vi "Read Graph Properties.vi"(0 "Config File":path, 7 "WFGraph Refnum":refnum<vi>, 9 "Section":string, 11 "error in (no error)":errorcluster) -> (4 "Config File out":path, 15 "error out":errorcluster)   [LabVIEW 2020]
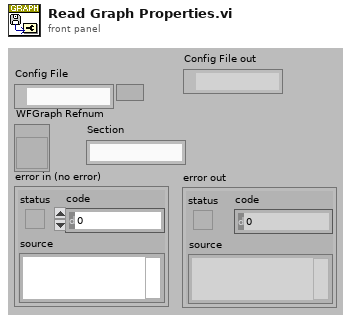
[diagram p1: front panel]
types:
  T1 = typedef "Graph Properties.ctl" = cluster{"X-axis":T2, "Y-axis":T2, "Plot Properties":T3[]}
  T2 = typedef "Axis Properties.ctl" = cluster{"Min":dbl, "Max":dbl, "Fit":u8}
  T3 = typedef "Plot Properties.ctl" = cluster{"Line Style":u8, "Line Width":u8, "Plot Color":u32, "Point Style":u8, "Point color":u32, "Interp":u8}
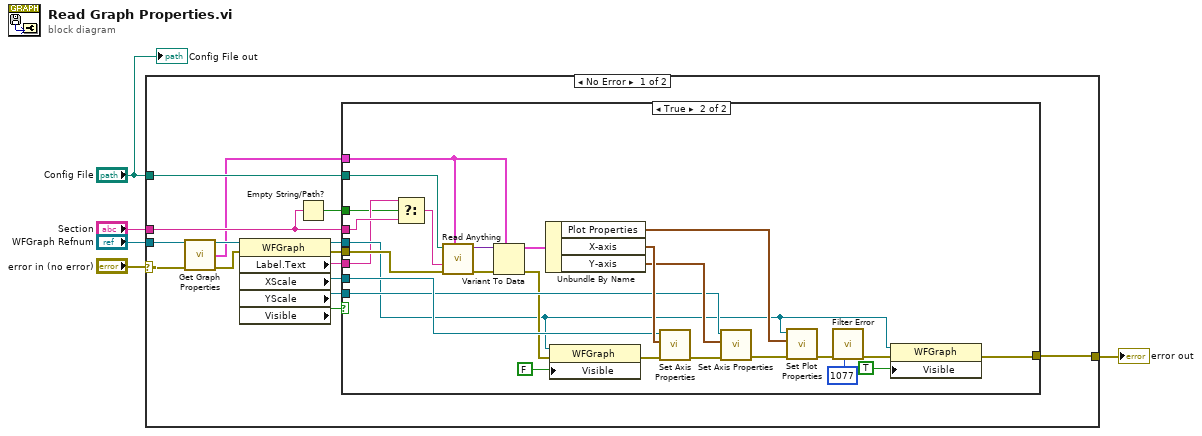
[diagram p0: block diagram]
diagram:
  n1 = case shown="No Error" "error in (no error)" {
    selector: "error in (no error)" -> [w10 w48]
    tunnel: "WFGraph Refnum" -> [w9 _]
    tunnel: "Config File" -> [w18 _]
    tunnel: [w13 w48] -> w2
    tunnel: "Section" -> [w12 _]
    frame No Error {
      n2 = call "Get Graph Properties.vi"("WFGraph Refnum"=w9, "error in (no error)"=w10) -> ("WFGraph Refnum (thru)"=w7:refnum<vi>, "Graph Properties"=w6:T1, "error out"=w8:errorcluster)  [unwired: 11 in]
      n3 = property class="WFGraph"(reference=w7, error in=w8) -> (reference out=w15:refnum<vi>, error out=w20:errorcluster, "Label.Text"=w19:string, "XScale"=w17:refnum<vi>, "YScale"=w16:refnum<vi>, "Visible"=w14:bool)
      n4 = Empty String/Path?(string/path=w12) -> (empty?=w11:bool)
      n5 = case shown="True" w14 {
        tunnel: w20 -> [w21 w46]
        tunnel: w19 -> [_ w23]
        tunnel: w18 -> [_ w45]
        tunnel: w6 -> [_ w42]
        tunnel: w17 -> [_ w38]
        tunnel: w16 -> [_ w36]
        tunnel: [w21 w30] -> w13
        tunnel: w15 -> [_ w27]
        tunnel: w12 -> [_ w25]
        tunnel: w11 -> [_ w22]
        frame False {
        }
        frame True {
          n6 = Select(t=w23, s=w22, f=w25) -> (s? t:f=w24:string)
          n7 = call "Read Anything.vi"("Type of Anything"=w42, "Error In"=w46, "Section Name (Name of \"Type of Anything\")"=w24, "Path (dialog)"=w45) -> ("Error Out"=w44:errorcluster, "Anything"=w43:variant)  [unwired: 5 in, 1 out]
          n8 = Variant To Data(error in=w44, type=w42, Variant=w43) -> (data=w40:T1, error out=w35:errorcluster)
          n9 = Unbundle By Name(w40) -> ("Plot Properties"=w34:T3[], "X-axis"=w39:T2, "Y-axis"=w37:T2)
          n10 = property class="WFGraph"(reference=w27, error in=w35, "Visible"=FALSE) -> (error out=w28:errorcluster)  [unwired: 1 out]
          n11 = call "Set Axis Properties.vi"("error in (no error)"=w28, "Axis Properties"=w39, "Scale Refnum"=w38) -> ("error out"=w47:errorcluster)  [unwired: 8 in]
          n12 = call "Set Axis Properties.vi"("error in (no error)"=w47, "Axis Properties"=w37, "Scale Refnum"=w36) -> ("error out"=w41:errorcluster)  [unwired: 8 in]
          n13 = call "Set Plot Properties.vi"("error in (no error)"=w41, "Plot Props"=w34, "Graph Refnum"=w27) -> ("error out"=w32:errorcluster)  [unwired: 8 in]
          n14 = call "Filter Error.vi"("error in (no error)"=w32, "code to ignore"=1077) -> ("error out"=w31:errorcluster)  [unwired: 9 in]
          n15 = property class="WFGraph"(reference=w27, error in=w31, "Visible"=TRUE ("Legend:Visible")) -> (error out=w30:errorcluster)  [unwired: 1 out]
        }
      }
    }
    frame Error {
    }
  }
  "error out" <- w2
  "Config File out" <- "Config File"
